vi "QueryServer_Start.vi"(7 "error in (no error)":errorcluster, 8 "Server Key File (.key)":path, 9 "Server Certificate File (.crt)":path, 10 "Server Address":string) -> (0 "error out":errorcluster, 2 "Event Registration Refnum":refnum<event-registration>, 3 "Server Info":T2)   [LabVIEW 2019, in "labview-grpc-query-server.lvlib"]
uses:
  labview-grpc-query-server.lvlib
  QueryServer_InvokeEventData.ctl
  VIs/grpcId.ctl
  VIs/MessageMetadata.ctl
  VIs/MessageElementMetadata.ctl
  VIs/MessageElementType.ctl
  VIs/gprc-support.lvlib
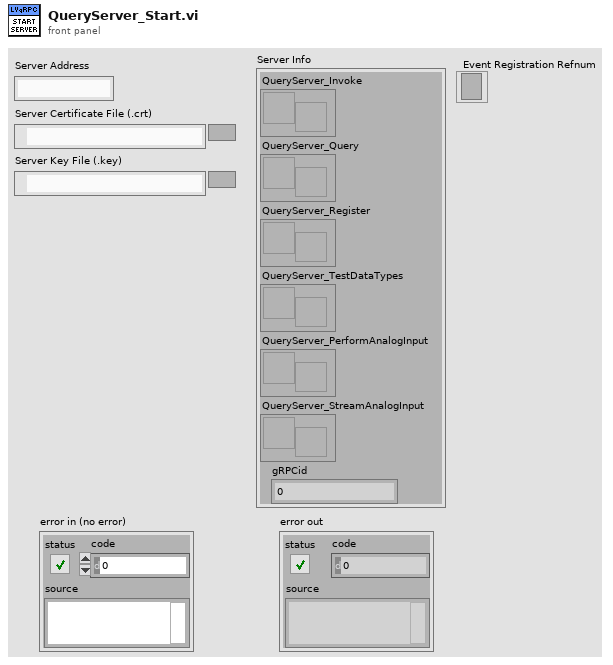
[diagram p1: front panel]
types:
  T1 = typedef "gprc-support.lvlib/grpcId.ctl" = u64
  T2 = cluster{"QueryServer_Invoke":refnum<user-event>, "QueryServer_Query":refnum<user-event>, "QueryServer_Register":refnum<user-event>, "QueryServer_TestDataTypes":refnum<user-event>, "QueryServer_PerformAnalogInput":refnum<user-event>, "QueryServer_StreamAnalogInput":refnum<user-event>, "gRPCid":T1}
  T3 = typedef "gprc-support.lvlib/MessageMetadata.ctl" = cluster{"Name":string, "Elements":T4[]}
  T4 = typedef "gprc-support.lvlib/MessageElementMetadata.ctl" = cluster{"Embedded Message Name":string, "Protobuf Index":i32, "MessageElementType":T5, "Repeated":bool}
  T5 = typedef "gprc-support.lvlib/MessageElementType.ctl" = enum32{"Int32Value", "FloatValue", "DoubleValue", "BoolValue", "StringValue", "MessageValue", ""}
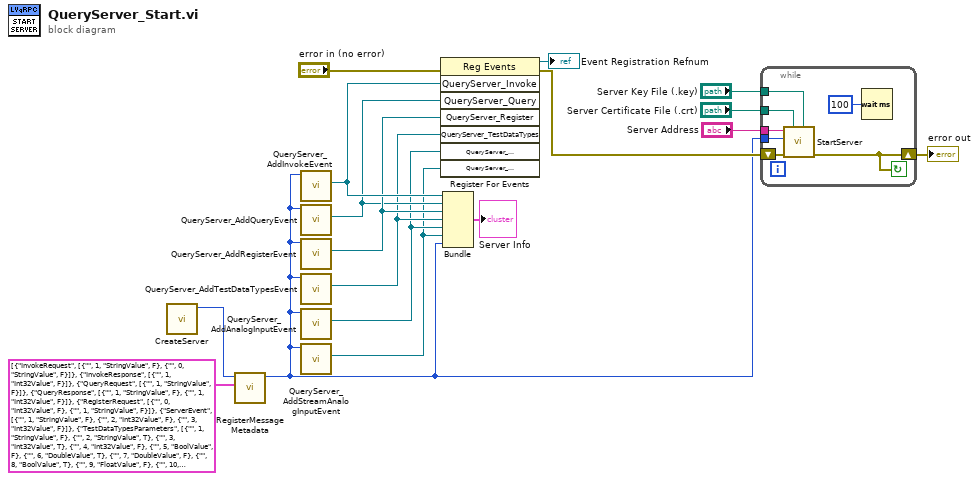
[diagram p0: block diagram]
diagram:
  n1 = call "CreateServer.vi"() -> ("gRPCid"=w12:T1)  [unwired: 11 in]
  n2 = call "RegisterMessageMetadata.vi"("Messages"=T3[] [{"Name"="InvokeRequest", "Elements"=[{"Embedded Message Name"="", "Protobuf Index"=1, "MessageElementType"=enum."StringValue", "Repeated"=FALSE}, {"Embedded Message Name"="", "Protobuf Index"=0, "MessageElementType"=enum."StringValue", "Repeated"=FALSE}]}, {"Name"="InvokeResponse", "Elements"=[{"Embedded Message Name"="", "Protobuf Index"=1, "MessageElementType"=enum."Int32Value", "Repeated"=FALSE}]}, {"Name"="QueryRequest", "Elements"=[{"Embedded Message Name"="", "Protobuf Index"=1, "MessageElementType"=enum."StringValue", "Repeated"=FALSE}]}, {"Name"="QueryResponse", "Elements"=[{"Embedded Message Name"="", "Protobuf Index"=1, "MessageElementType"=enum."StringValue", "Repeated"=FALSE}, {"Embedded Message Name"="", "Protobuf Index"=1, "MessageElementType"=enum."Int32Value", "Repeated"=FALSE}]}, {"Name"="RegisterRequest", "Elements"=[{"Embedded Message Name"="", "Protobuf Index"=0, "MessageElementType"=enum."Int32Value", "Repeated"=FALSE}, {"Embedded Message Name"="", "Protobuf Index"=1, "MessageElementType"=enum."StringValue", "Repeated"=FALSE}]}, {"Name"="ServerEvent", "Elements"=[{"Embedded Message Name"="", "Protobuf Index"=1, "MessageElementType"=enum."StringValue", "Repeated"=FALSE}, {"Embedded Message Name"="", "Protobuf Index"=2, "MessageElementType"=enum."Int32Value", "Repeated"=FALSE}, {"Embedded Message Name"="", "Protobuf Index"=3, "MessageElementType"=enum."Int32Value", "Repeated"=FALSE}]}, {"Name"="TestDataTypesParameters", "Elements"=[{"Embedded Message Name"="", "Protobuf Index"=1, "MessageElementType"=enum."StringValue", "Repeated"=FALSE}, {"Embedded Message Name"="", "Protobuf Index"=2, "MessageElementType"=enum."StringValue", "Repeated"=TRUE}, {"Embedded Message Name"="", "Protobuf Index"=3, "MessageElementType"=enum."Int32Value", "Repeated"=TRUE}, {"Embedded Message Name"="", "Protobuf Index"=4, "MessageElementType"=enum."Int32Value", "Repeated"=FALSE}, {"Embedded Message Name"="", "Protobuf Index"=5, "MessageElementType"=enum."BoolValue", "Repeated"=FALSE}, {"Embedded Message Name"="", "Protobuf Index"=6, "MessageElementType"=enum."DoubleValue", "Repeated"=TRUE}, {"Embedded Message Name"="", "Protobuf Index"=7, "MessageElementType"=enum."DoubleValue", "Repeated"=FALSE}, {"Embedded Message Name"="", "Protobuf Index"=8, "MessageElementType"=enum."BoolValue", "Repeated"=TRUE}, {"Embedded Message Name"="", "Protobuf Index"=9, "MessageElementType"=enum."FloatValue", "Repeated"=FALSE}, {"Embedded Message Name"="", "Protobuf Index"=10, "MessageElementType"=enum."FloatValue", "Repeated"=TRUE}, {"Embedded Message Name"="DataTypeTest", "Protobuf Index"=11, "MessageElementType"=enum."MessageValue", "Repeated"=FALSE}, {"Embedded Message Name"="DataTypeTest", "Protobuf Index"=12, "MessageElementType"=enum."MessageValue", "Repeated"=TRUE}]}, {"Name"="DataTypeTest", "Elements"=[{"Embedded Message Name"="", "Protobuf Index"=1, "MessageElementType"=enum."BoolValue", "Repeated"=FALSE}, {"Embedded Message Name"="", "Protobuf Index"=2, "MessageElementType"=enum."Int32Value", "Repeated"=FALSE}, {"Embedded Message Name"="", "Protobuf Index"=3, "MessageElementType"=enum."FloatValue", "Repeated"=FALSE}, {"Embedded Message Name"="", "Protobuf Index"=4, "MessageElementType"=enum."DoubleValue", "Repeated"=FALSE}]}, {"Name"="AnalogInputRequest", "Elements"=[]}, {"Name"="AnalogInputData", "Elements"=[{"Embedded Message Name"="", "Protobuf Index"=1, "MessageElementType"=enum."FloatValue", "Repeated"=TRUE}, {"Embedded Message Name"="", "Protobuf Index"=2, "MessageElementType"=enum."FloatValue", "Repeated"=TRUE}, {"Embedded Message Name"="", "Protobuf Index"=3, "MessageElementType"=enum."FloatValue", "Repeated"=TRUE}, {"Embedded Message Name"="", "Protobuf Index"=4, "MessageElementType"=enum."FloatValue", "Repeated"=TRUE}, {"Embedded Message Name"="", "Protobuf Index"=5, "MessageElementType"=enum."FloatValue", "Repeated"=TRUE}, {"Embedded Message Name"="", "Protobuf Index"=6, "MessageElementType"=enum."FloatValue", "Repeated"=TRUE}, {"Embedded Message Name"="", "Protobuf Index"=7, "MessageElementType"=enum."FloatValue", "Repeated"=TRUE}, {"Embedded Message Name"="", "Protobuf Index"=8, "MessageElementType"=enum."FloatValue", "Repeated"=TRUE}, {"Embedded Message Name"="", "Protobuf Index"=9, "MessageElementType"=enum."FloatValue", "Repeated"=TRUE}, {"Embedded Message Name"="", "Protobuf Index"=10, "MessageElementType"=enum."StringValue", "Repeated"=FALSE}, {"Embedded Message Name"="", "Protobuf Index"=11, "MessageElementType"=enum."FloatValue", "Repeated"=FALSE}, {"Embedded Message Name"="", "Protobuf Index"=12, "MessageElementType"=enum."BoolValue", "Repeated"=FALSE}, {"Embedded Message Name"="", "Protobuf Index"=13, "MessageElementType"=enum."Int32Value", "Repeated"=FALSE}, {"Embedded Message Name"="", "Protobuf Index"=14, "MessageElementType"=enum."StringValue", "Repeated"=FALSE}]}], "gRPCid"=w12) -> ("gRPCid"=w4:T1)  [unwired: 8 in, 1 out]
  n3 = call "QueryServer_AddInvokeEvent.vi"("gRPCid in"=w4) -> ("QueryServer_Invoke"=w16:refnum<user-event>)  [unwired: 9 in, 1 out]
  n4 = call "QueryServer_AddQueryEvent.vi"("gRPCid in"=w4) -> ("QueryServer_Query"=w14:refnum<user-event>)  [unwired: 9 in, 1 out]
  n5 = call "QueryServer_AddRegisterEvent.vi"("gRPCid in"=w4) -> ("QueryServer_Register"=w15:refnum<user-event>)  [unwired: 9 in, 1 out]
  n6 = call "QueryServer_AddTestDataTypesEvent.vi"("gRPCid in"=w4) -> ("QueryServer_TestDataTypes"=w13:refnum<user-event>)  [unwired: 9 in, 1 out]
  n7 = call "QueryServer_AddAnalogInputEvent.vi"("gRPCid in"=w4) -> ("QueryServer_PerformAnalogInput"=w5:refnum<user-event>)  [unwired: 9 in, 1 out]
  n8 = call "QueryServer_AddStreamAnalogInputEvent.vi"("gRPCid in"=w4) -> ("QueryServer_StreamAnalogInput"=w3:refnum<user-event>)  [unwired: 9 in, 1 out]
  n9 = register-events(error in="error in (no error)", w16, w14, w15, w13, w5, w3) -> (reference out=→"Event Registration Refnum":refnum<event-registration>, error out=w9:errorcluster)  [unwired: 1 in]
  n10 = Bundle("QueryServer_Invoke"=w16, "QueryServer_Query"=w14, "QueryServer_Register"=w15, "QueryServer_TestDataTypes"=w13, "QueryServer_PerformAnalogInput"=w5, "QueryServer_StreamAnalogInput"=w3, "gRPCid"=w4) -> (→"Server Info":T2)  [unwired: 1 in]
  n11 = while {
    tunnel: w4 -> [w24]
    tunnel: "Server Address" -> [w22]
    tunnel: "Server Certificate File (.crt)" -> [w21]
    tunnel: "Server Key File (.key)" -> [w20]
    shift-right: [w18] -> w10
    shift-left: w9 -> [w23]
    stop <- w18 continue-if-true
    n12 = call "StartServer.vi"("Server Key File (.key)"=w20, "Server Certificate File (.crt)"=w21, "error in (no error)"=w23, "gRPCid"=w24, "Server Address"=w22) -> ("error out"=w18:errorcluster)  [unwired: 6 in]
    n13 = Wait (ms)(milliseconds to wait=u32 100) -> ()  [unwired: 1 out]
  }
  "error out" <- w10
